vi "LRU Stop.vi"   [LabVIEW 2019, in "23.lvlib"]
uses:
  23.lvlib
types:
  T1 = cluster{"Stop":bool, "Check":bool, "Key":cluster{"Hallway":string[], "Rooms":string[][]}, "Value":u64, "Check Notifier":refnum<notifier>}
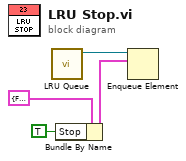
[diagram p0: block diagram]
diagram:
  n1 = call "LRU Queue.vi"() -> ("LRU Queue"=w2:refnum<queue>)  [unwired: 11 in]
  n2 = Bundle By Name(cluster=T1 {"Stop"=FALSE, "Check"=FALSE, "Key"={"Hallway"=[], "Rooms"=[]}, "Value"=0, "Check Notifier"=refnum}, "Stop"=TRUE) -> (w3:T1)
  n3 = Enqueue Element(queue=w2, element=w3) -> ()  [unwired: 2 in, 3 out]
